vi "Initial Password.vi"(8 "error in (no error)":errorcluster, 11 "Masterv2 in":refnum<class "Masterv2.lvclass">) -> (0 "error out":errorcluster, 3 "Masterv2 out":refnum<class "Masterv2.lvclass">)   [LabVIEW 2014, in "Main Libraryv2.lvlib" / "Masterv2.lvclass"]
uses:
  Master/Masterv2.lvclass
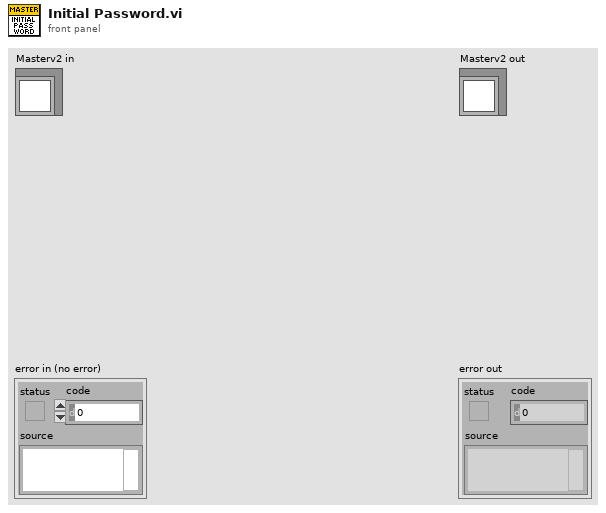
[diagram p1: front panel]
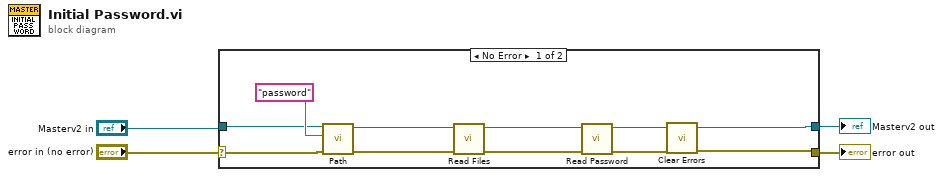
[diagram p0: block diagram]
diagram:
  n1 = case shown="No Error" "error in (no error)" {
    selector: "error in (no error)" -> [w14 w16]
    tunnel: [w5 w16] -> w3
    tunnel: [w7 w15] -> w1
    tunnel: "Masterv2 in" -> [w10 w15]
    frame No Error {
      n2 = call-dynamic "Path.vi"("error in (no error)"=w14, "pathname"="password", "Masterv2 in"=w10) -> ("error out"=w13:errorcluster, "Masterv2 out"=w9:refnum<class "Masterv2.lvclass">)  [unwired: 7 in]
      n3 = call-dynamic "Read Files.vi"("error in (no error)"=w13, "Masterv2 in"=w9) -> ("error out"=w12:errorcluster, "Masterv2 out"=w8:refnum<class "Masterv2.lvclass">)  [unwired: 8 in]
      n4 = call-dynamic "Read Password.vi"("error in (no error)"=w12, "Masterv2 in"=w8) -> ("error out"=w6:errorcluster, "Masterv2 out"=w7:refnum<class "Masterv2.lvclass">)  [unwired: 8 in]
      n5 = call <vilib>:"Clear Errors.vi"("error in (no error)"=w6) -> ("error out"=w5:errorcluster)  [unwired: 5 in, 1 out]
    }
    frame Error {
    }
  }
  "error out" <- w3
  "Masterv2 out" <- w1
